vi "Pixel2Pos.vi"(10 "Secondary":i32, 11 "Primary":i32) -> (3 "Position (m)":cluster{"X":dbl, "\nY":dbl, "\nZ":dbl})   [LabVIEW 2016]
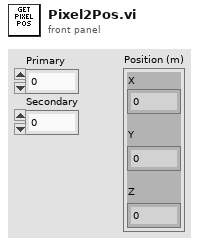
[diagram p1: front panel]
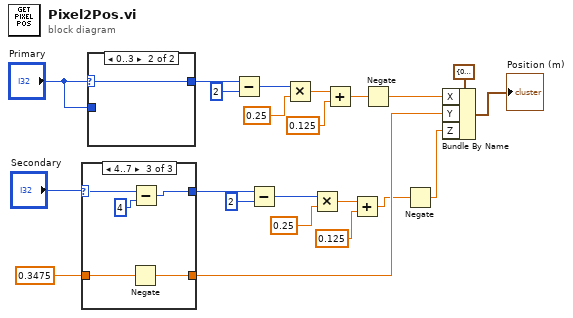
[diagram p0: block diagram]
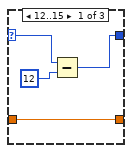
[diagram p2: hidden frame]
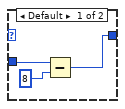
[diagram p4: hidden frame]
diagram:
  n1 = case shown="4..7" "Secondary" {
    selector: "Secondary" -> [w24 w28 w33]
    tunnel: [w25 w28 w31] -> w9
    tunnel: 0.3475 -> [w23 w27 w30]
    tunnel: [w23 w27 w29] -> w3
    frame 12..15 {
      n2 = Subtract(x=w24, y=12) -> (x-y=w25:i32)
    }
    frame Default {
    }
    frame 4..7 {
      n3 = Negate(x=w30) -> (-x=w29:dbl)
      n4 = Subtract(x=w33, y=4) -> (x-y=w31:i32)
    }
  }
  n5 = case shown="0..3" "Primary" {
    selector: "Primary" -> [_ w37]
    tunnel: "Primary" -> [w36 _]
    tunnel: [w34 w37] -> w18
    frame Default {
      n6 = Subtract(x=w36, y=8) -> (x-y=w34:i32)
    }
    frame 0..3 {
    }
  }
  n7 = Subtract(x=w18, y=2) -> (x-y=w16:i32)
  n8 = Subtract(x=w9, y=2) -> (x-y=w14:i32)
  n9 = Multiply(x=w16, y=0.25) -> (x*y=w20:dbl)
  n10 = Multiply(x=w14, y=0.25) -> (x*y=w11:dbl)
  n11 = Add(x=w20, y=0.125) -> (x+y=w8:dbl)
  n12 = Add(x=w11, y=0.125) -> (x+y=w2:dbl)
  n13 = Negate(x=w8) -> (-x=w5:dbl)
  n14 = Negate(x=w2) -> (-x=w1:dbl)
  n15 = Bundle By Name(cluster=cluster{"X":dbl, "\nY":dbl, "\nZ":dbl} {"X"=0.0, "\nY"=0.0, "\nZ"=0.0}, "X"=w5, "Y"=w3, "Z"=w1) -> (→"Position (m)":cluster{"X":dbl, "\nY":dbl, "\nZ":dbl})
